vi "StartAllHardWare.vi"(8 "entrée d'erreur (pas d'erreur)":errorcluster, 10 "ON/OFF":bool, 11 "Control en entrée":refnum<class "Control-Server.lvclass">) -> (0 "sortie d'erreur":errorcluster, 3 "Control en sortie":refnum<class "Control-Server.lvclass">)   [LabVIEW 2018, in "Control-Server.lvclass"]
uses:
  Classes/Control/Control-Server/Control-Server.lvclass
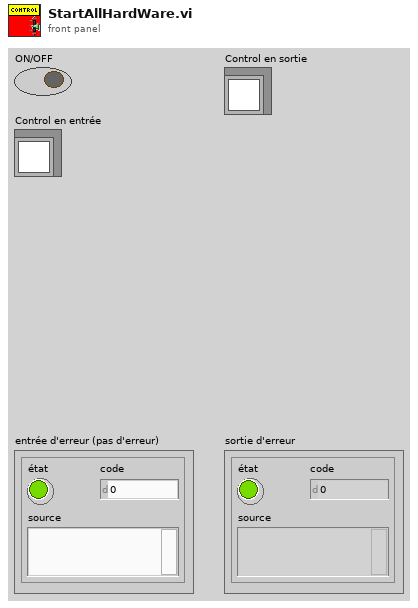
[diagram p1: front panel]
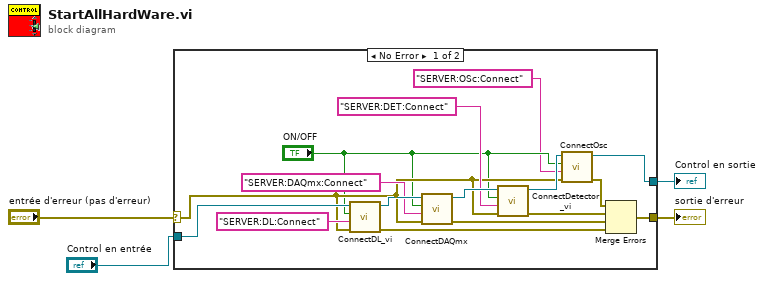
[diagram p0: block diagram]
diagram:
  n1 = case shown="No Error" "entrée d'erreur (pas d'erreur)" {
    selector: "entrée d'erreur (pas d'erreur)" -> [w7 w21]
    tunnel: "Control en entrée" -> [w20 w22]
    tunnel: [w9 w22] -> w3
    tunnel: [w14 w21] -> w2
    frame No Error {
      n2 = call "ConnectDL_vi.vi"("error in (no error)"=w7, "Command"="SERVER:DL:Connect", "ON/OFF"="ON/OFF", "Control in"=w20) -> ("error out"=w16:errorcluster, "Control out"=w18:refnum<class "Control-Server.lvclass">)  [unwired: 6 in]
      n3 = call "ConnectDAQmx.vi"("error in"=w7, "Command"="SERVER:DAQmx:Connect", "ON/OFF"="ON/OFF", "Control in"=w18) -> ("error out"=w15:errorcluster, "Control out"=w19:refnum<class "Control-Server.lvclass">)  [unwired: 6 in]
      n4 = call "ConnectDetector_vi.vi"("error in (no error)"=w7, "Command"="SERVER:DET:Connect", "ON/OFF"="ON/OFF", "Control in"=w19) -> ("error out"=w17:errorcluster, "Control out"=w10:refnum<class "Control-Server.lvclass">)  [unwired: 6 in]
      n5 = call "ConnectOsc.vi"("error in (no error)"=w7, "Command"="SERVER:OSc:Connect", "ON/OFF"="ON/OFF", "Control in"=w10) -> ("error out"=w8:errorcluster, "Control out"=w9:refnum<class "Control-Server.lvclass">)  [unwired: 6 in]
      n6 = Merge Errors(w8, w17, w15, w16) -> (w14:errorcluster)
    }
    frame Error {
    }
  }
  "sortie d'erreur" <- w2
  "Control en sortie" <- w3
